vi "Speichern in Datei.vi"(4 "delimiter (\\t)":string="\t" caption="Trennzeichen (\\t)", 5 "format (%s)":string="%s" caption="Format (%s)", 6 "transpose? (no:F)":bool caption="Transponieren? (nein:F)", 8 "append to file? (new file:F)":bool caption="An Datei anhängen? (Neue Datei:F)", 9 "1D data":string[](array[string]) caption="1D-Daten", 10 "2D data":string[][](array[string]) caption="2D-Daten", 11 "file path (dialog if empty)":path caption="Dateipfad (Dialog, wenn leer)") -> (0 "error out":errorcluster caption="Fehler (Ausgang)", 3 "new file path (Not A Path if cancelled)":path caption="Neuer Dateipfad (Kein Pfad, wenn abgebrochen)")   [LabVIEW 2020, in "LogKonfig.lvlib"]
uses:
  LogKonfig.lvlib
panel:
  in  "prompt":string="Datei zum Schreiben auswählen." caption="Eingabeaufforderung"
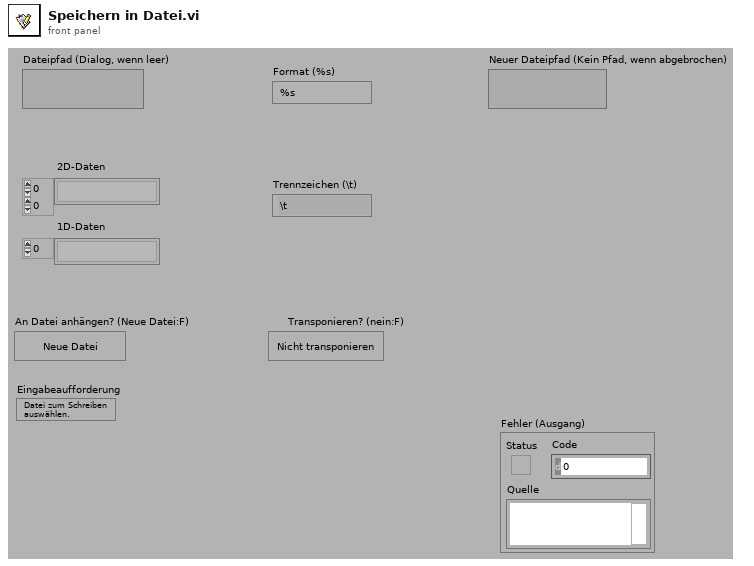
[diagram p1: front panel]
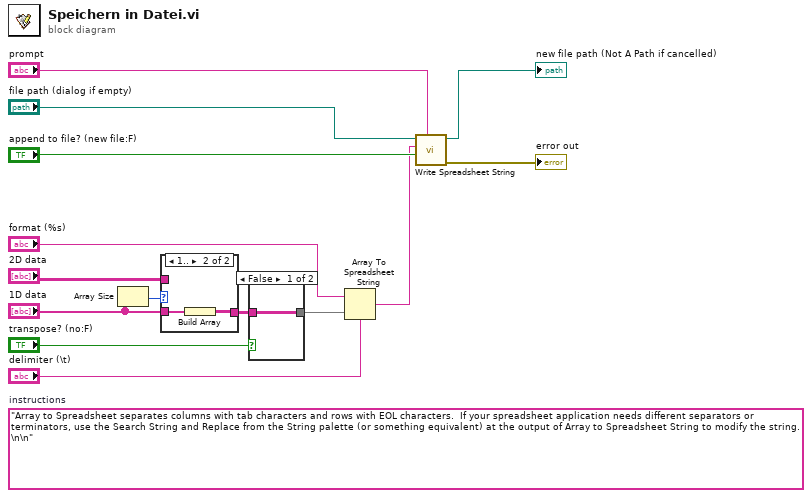
[diagram p0: block diagram]
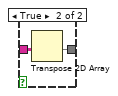
[diagram p2: hidden frame]
diagram:
  (unwired) "Array to Spreadsheet separates columns with tab characters and rows with EOL characters.  If your spreadsheet application needs different separators or terminators, use the Search String and Replace from the String palette (or something equivalent) at the output of Array to Spreadsheet String to modify the string.\n\n"  # instructions
  n1 = Array Size(array="1D data") -> (size(s)=w14:i32)
  n2 = case shown="1.." w14 {
    tunnel: "1D data" -> [_ w17]
    tunnel: [w15 w16] -> w10
    tunnel: "2D data" -> [w15 _]
    frame ..0 {
      # "1D array is empty"
    }
    frame 1.. {
      n3 = Build Array(w17) -> (w16:string[][])
    }
  }
  n4 = case shown="False" "transpose? (no:F)" {
    tunnel: [w18 w20] -> w8
    tunnel: w10 -> [w18 w19]
    frame False {
    }
    frame True {
      n5 = Transpose 2D Array(2D array=w19) -> (transposed array=w20:string[][])
    }
  }
  n6 = Array To Spreadsheet String(delimiter (Tab)="delimiter (\\t)", array=w8, 3:"format (%s)") -> (spreadsheet string=w2:string)
  n7 = call <vilib>:"Write Spreadsheet String.vi"("prompt"="prompt", "append to file? (new file:F)"="append to file? (new file:F)", "spreadsheet string"=w2, "file path (dialog if empty)"="file path (dialog if empty)") -> ("error out"=→"error out":errorcluster, "path"=→"new file path (Not A Path if cancelled)":path)  [unwired: 6 in]
